vi "FlowRateValidation.vi"(0 "GEA2 Reference In":refnum<k24>, 1 "GEA Inputs":T4 {"Destination" format="%.0x"; "Source" format="%.0x"}, 11 "Error In":errorcluster, 12 "Repeat Count":i32, 13 "Read ERD List":T2[](array[typedef]) {"ERD Number" format="%.0x"}) -> (4 "GEA2 Reference Out":refnum<k24>, 8 "ERD Data Out":T1[](array[typedef]) {"ERD Number" format="%.0x"}, 10 "Raw Data Out":string, 15 "Error Out":errorcluster)   [LabVIEW 2016, in "TL27.lvlib"]
doc: "This vi can be used to read ERD every 1 sec for user selected repeat counts."
uses:
  Projects/TL27.lvlib
  C:/Automation/DLLs/PC Dot Net/GeaCommunication.dll
  Common/LabVIEW GEA2 Toolkit/LabVIEW_GEA2_Toolkit.lvlibp/type defs/Source_Destination.ctl
  Common/LabVIEW GEA2 Toolkit/LabVIEW_GEA2_Toolkit.lvlibp/type defs/ERD Read Data In.ctl
  Common/LabVIEW GEA2 Toolkit/LabVIEW_GEA2_Toolkit.lvlibp/type defs/Data Type.ctl
  Common/LabVIEW GEA2 Toolkit/LabVIEW_GEA2_Toolkit.lvlibp/type defs/ERD Read Data Out.ctl
  Common/LabVIEW GEA2 Toolkit/LabVIEW_GEA2_Toolkit.lvlibp
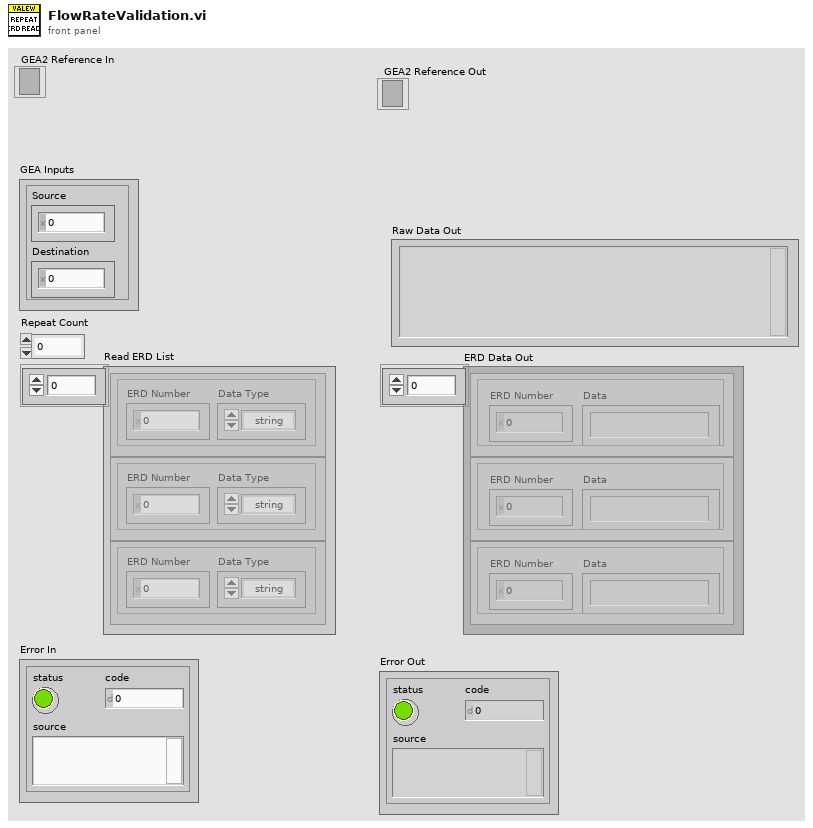
[diagram p1: front panel]
types:
  T1 = typedef "LabVIEW_GEA2_Toolkit.lvlibp/ERD Read Data Out.ctl" = cluster{"ERD Number":u16, "Data":string}
  T2 = typedef "LabVIEW_GEA2_Toolkit.lvlibp/ERD Read Data In.ctl" = cluster{"ERD Number":u16, "Data Type":T3}
  T3 = typedef "LabVIEW_GEA2_Toolkit.lvlibp/Data Type.ctl" = enum16{"string", "boolean", "uint8_t", "uint16_t", "uint32_t", "uint64_t", "int8_t", "int16_t", "int32_t", "int64_t"}
  T4 = typedef "LabVIEW_GEA2_Toolkit.lvlibp/Source_Destination.ctl" = cluster{"Source":u8, "Destination":u8}
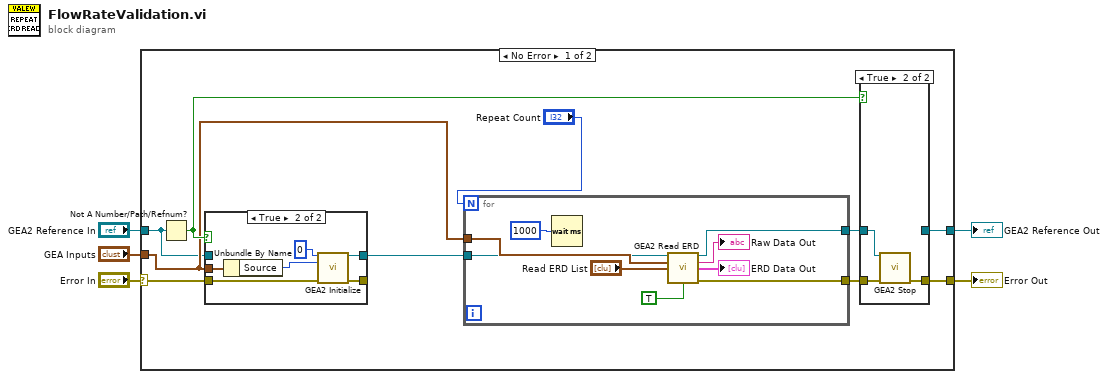
[diagram p0: block diagram]
diagram:
  n1 = case shown="No Error" "Error In" {
    selector: "Error In" -> [w9 w38]
    tunnel: "GEA Inputs" -> [w11 _]
    tunnel: "GEA2 Reference In" -> [w10 w39]
    tunnel: [w8 w39] -> w2
    tunnel: [w7 w38] -> w1
    frame No Error {
      n2 = Not A Number/Path/Refnum?(number/path/refnum=w10) -> (NaN/Path/Refnum?=w12:bool)
      n3 = case shown="True" w12 {
        tunnel: w9 -> [w31 w37]
        tunnel: [w31 w36] -> _
        tunnel: [w30 w35] -> w6
        tunnel: w11 -> [_ w33]
        tunnel: w10 -> [w30 _]
        frame False {
        }
        frame True {
          n4 = Unbundle By Name(w33) -> ("Source"=w34:u8)
          n5 = call "GEA2 Initialize.vi"("Board Index"=0, "Source Address"=w34, "error in"=w37) -> ("GEA2 Reference Out"=w35:refnum<k24>, "error out"=w36:errorcluster)  [unwired: 10 in, 1 out]
        }
      }
      n6 = for {
        N: "Repeat Count" -> [_]
        tunnel: w11 -> [w24]
        tunnel: [w18] -> w14
        tunnel: [w23] -> w13
        tunnel: w6 -> [w16]
        n7 = Wait (ms)(milliseconds to wait=u32 1000) -> ()  [unwired: 1 out]
        n8 = call "GEA2 Read ERD.vi"("GEA2 Reference In"=w16, "GEA Inputs"=w24, "Read ERD List"="Read ERD List", "Verify ERD Response?"=TRUE) -> ("GEA2 Reference Out"=w23:refnum<k24>, "Raw Data Out"=→"Raw Data Out":string, "ERD Data Out"=→"ERD Data Out":T1[], "Error Out"=w18:errorcluster)  [unwired: 8 in]
      }
      n9 = case shown="True" w12 {
        tunnel: w14 -> [w25 w28]
        tunnel: [w25 w27] -> w7
        tunnel: w13 -> [w26 w29]
        tunnel: [w26 _] -> w8
        frame False {
        }
        frame True {
          n10 = call "GEA2 Stop.vi"("GEA2 Reference In"=w29, "Error In"=w28) -> ("Error Out"=w27:errorcluster)  [unwired: 13 in]
        }
      }
    }
    frame Error {
    }
  }
  "GEA2 Reference Out" <- w2
  "Error Out" <- w1
